vi "HTTP Server.vi"(8 "error in (no error)":errorcluster, 11 "GodotServer in":refnum<class "GodotServer.lvclass">) -> (0 "error out":errorcluster, 2 "HTTP Server":refnum<class "Server.lvclass">, 3 "GodotServer out":refnum<class "GodotServer.lvclass">)   [LabVIEW 2020, in "GodotLV.lvlib" / "GodotServer.lvclass"]
uses:
  GodotServer.lvclass
  <vilib>/IlluminatedG/IG HTTP Server/HTTP Server/Server/Server.lvclass
  GodotServer.lvclass/GodotServer.ctl
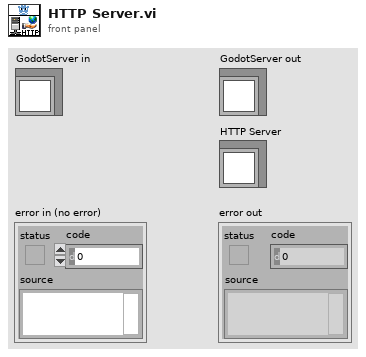
[diagram p1: front panel]
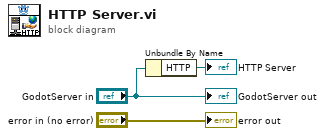
[diagram p0: block diagram]
diagram:
  n1 = Unbundle By Name("GodotServer in") -> ("HTTP"=→"HTTP Server":refnum<class "Server.lvclass">)
  "error out" <- "error in (no error)"
  "GodotServer out" <- "GodotServer in"
